vi "Check SSH Connection Status.vi"(8 "Error In":errorcluster, 11 "Install LV Data in":T1={"SSH Session"=refnum, "Status Log"="", "Detailed Log"="", "Credentials"={"Hostname or IP"="192.168.7.2", "Username"="root", "Password"=""}, "Target Info"={"OS Version"="", "CPU"="", "Systemd Version"="", "Internet Access"=FALSE, "Device Type"="", "LV Installed Ver"="", "LV Available Ver"="", "LV Upgrade Available"=FALSE, "Hostname"="", "NIC Info"=[]}, "Reboot Required?"=FALSE}) -> (0 "Error Out":errorcluster, 2 "IsConnected":bool, 3 "Install LV Data":T1={"SSH Session"=refnum, "Status Log"="", "Detailed Log"="", "Credentials"={"Hostname or IP"="192.168.7.2", "Username"="root", "Password"=""}, "Target Info"={"OS Version"="", "CPU"="", "Systemd Version"="", "Internet Access"=FALSE, "Device Type"="", "LV Installed Ver"="", "LV Available Ver"="", "LV Upgrade Available"=FALSE, "Hostname"="", "NIC Info"=[]}, "Reboot Required?"=FALSE})   [LabVIEW 2020, in "LMH-LINX.lvlib"]
uses:
  LMH-LINX.lvlib
  C:/Users/rkalbermatter/Projects/LabVIEW Hobbyist/LabVIEW/vi.lib/MakerHub/LINX/Resources/Renci.SshNet.dll
  Projects/LabVIEW Hobbyist/LabVIEW/vi.lib/MakerHub/LINX/Resources/Renci.SshNet.dll
  SSH/SSH Unix Session Op.ctl
  Target Info.ctl
  Install LV Data.ctl
  NIC Info.ctl
  NIC Mode.ctl
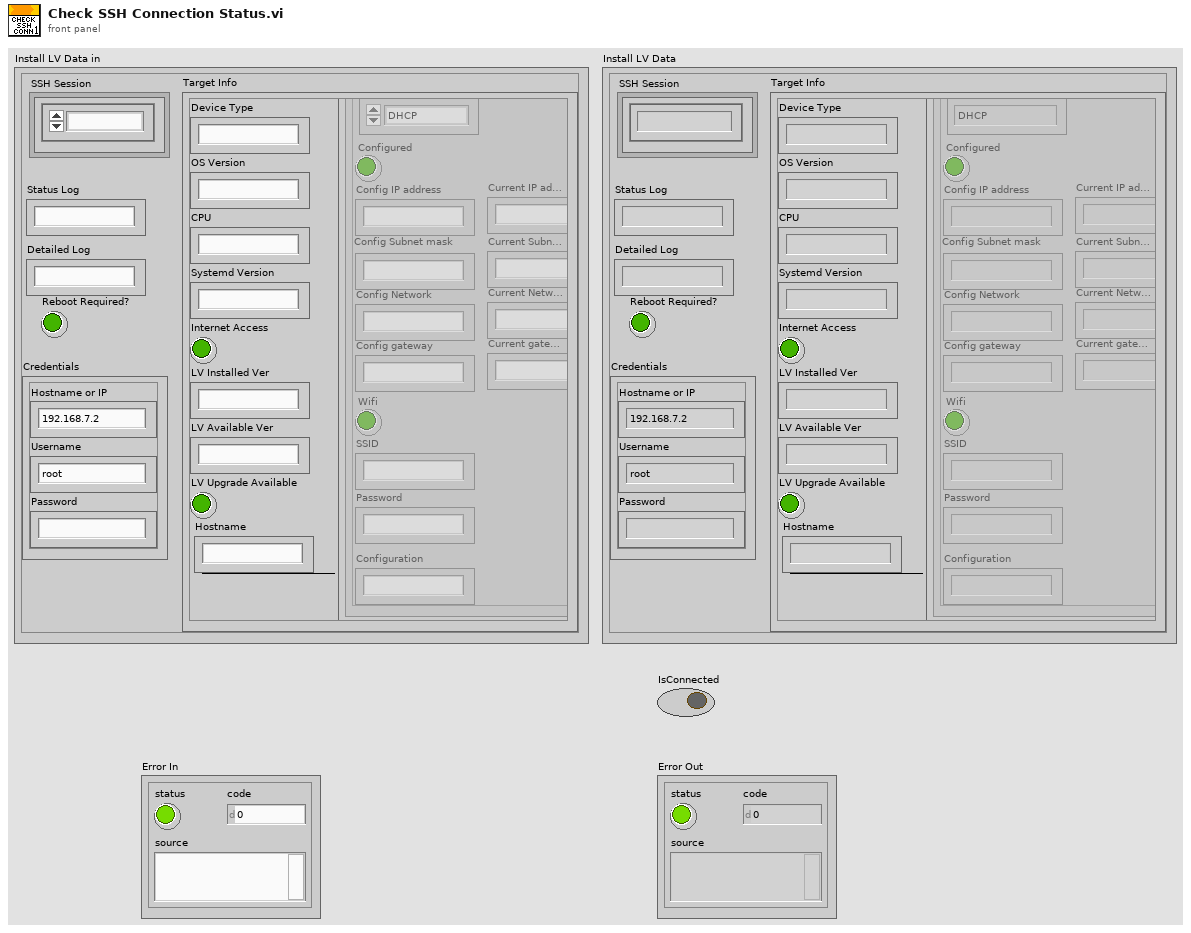
[diagram p1: front panel]
types:
  T1 = typedef "LMH-LINX.lvlib/Install LV Data.ctl" = cluster{"SSH Session":refnum<k1>, "Status Log":string, "Detailed Log":string, "Credentials":cluster{"Hostname or IP":string, "Username":string, "Password":string}, "Target Info":T2, "Reboot Required?":bool}
  T2 = typedef "LMH-LINX.lvlib/Target Info.ctl" = cluster{"OS Version":string, "CPU":string, "Systemd Version":string, "Internet Access":bool, "Device Type":string, "LV Installed Ver":string, "LV Available Ver":string, "LV Upgrade Available":bool, "Hostname":string, "NIC Info":T3[]}
  T3 = typedef "LMH-LINX.lvlib/NIC Info.ctl" = cluster{"Name":string, "NIC Mode":T4, "Configured":bool, "Config IP address":string, "Config Subnet mask":string, "Config Network":string, "Config gateway":string, "Wifi":bool, "SSID":string, "Password":string, "Configuration":string, "Current IP address":string, "Current Subnet mask":string, "Current gateway":string, "Current Network":string}
  T4 = typedef "LMH-LINX.lvlib/NIC Mode.ctl" = enum16{"DHCP", "Static", "Loopback"}
  T5 = typedef "LMH-LINX.lvlib/SSH Unix Session Op.ctl" = enum16{"New", "Get", "Delete"}
  T6 = typedef "LMH-LINX.lvlib/SSH Unix Session Info.ctl" = cluster{"PID":i32, "Read FD":i32, "Write FD":i32, "Error FD":i32}
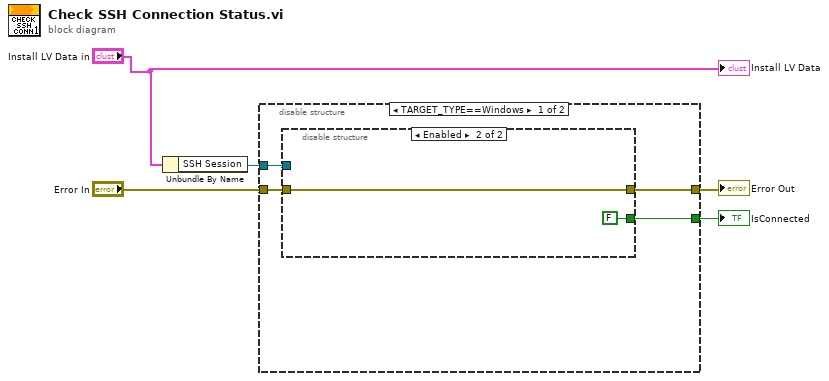
[diagram p0: block diagram]
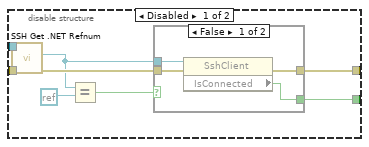
[diagram p2: hidden frame]
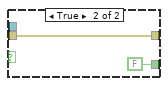
[diagram p3: hidden frame]
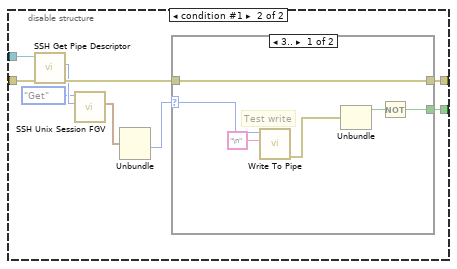
[diagram p4: hidden frame]
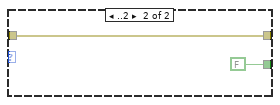
[diagram p5: hidden frame]
diagram:
  n1 = Unbundle By Name("Install LV Data in") -> ("SSH Session"=w1:refnum<k1>)
  n2 = disable-structure shown="TARGET_TYPE==Windows" {
    disable-tunnel: [w9 w34] -> w5
    disable-tunnel: [w8 w33] -> w4
    disable-tunnel: "Error In" -> [w7 w32]
    disable-tunnel: w1 -> [w6 w31]
    frame condition #0 (active) {
      n3 = disable-structure shown="Enabled" {
        disable-tunnel: [w17 FALSE ("IsConnected")] -> w9
        disable-tunnel: [w16 w25] -> w8
        disable-tunnel: w7 -> [w15 w25]
        disable-tunnel: w6 -> [w14 _]
        frame Disabled {
          n4 = call "SSH Get .NET Refnum.vi"("Error In"=w15, "SSH Session"=w14) -> ("Error Out"=w12:errorcluster, "SSH .NET Refnum"=w11:refnum<k24>)  [unwired: 7 in, 1 out]
          n5 = Equal?(x=w11, y=refnum<k0> refnum) -> (x = y?=w10:bool)
          n6 = case shown="False" w10 {
            tunnel: [w21 FALSE ("IsConnected")] -> w17
            tunnel: [w20 w22] -> w16
            tunnel: w12 -> [w19 w22]
            tunnel: w11 -> [w18 _]
            frame False {
              n7 = property class="SshClient"(reference=w18, error in=w19) -> (error out=w20:errorcluster, "IsConnected"=w21:bool)  [unwired: 1 out]
            }
            frame True {
            }
          }
        }
        frame Enabled {
        }
      }
    }
    frame condition #1 {
      n8 = call "SSH Get Pipe Descriptor.vi"("Error In"=w32, "SSH Session"=w31) -> ("Error Out"=w30:errorcluster, "SSH Pipe Descriptor"=w29:i32)  [unwired: 7 in, 1 out]
      n9 = call "SSH Unix Session FGV.vi"("Session In"=w29, "Operation"=SSH_Unix_Session_Op."Get") -> ("info in"=w27:T6)  [unwired: 8 in, 1 out]
      n10 = Unbundle(w27) -> ("Write FD"=w26:i32)  [unwired: 3 out]
      n11 = case shown="3.." w26 {
        selector: w26 -> [w39 _]
        tunnel: [w36 FALSE ("IsConnected")] -> w34
        tunnel: [w35 w41] -> w33
        tunnel: w30 -> [w35 w41]
        frame 3.. {
          # "Test write"
          n12 = call <vilib>:"Write To Pipe.vi"("data"="\n", "file descriptor"=w39) -> ("error out"=w38:errorcluster)  [unwired: 3 in, 2 out]
          n13 = Unbundle(w38) -> ("status"=w37:bool)  [unwired: 2 out]
          n14 = Not(x=w37) -> (.not. x?=w36:bool)
        }
        frame ..2 {
        }
      }
    }
  }
  "IsConnected" <- w5
  "Error Out" <- w4
  "Install LV Data" <- "Install LV Data in"
